vi "Slewing Test.vi"(8 "error in (no error)":errorcluster, 10 "Model in":refnum<class "Model.lvclass">, 11 "Test Actuator State in":refnum<class "Test Actuator State.lvclass">) -> (0 "error out":errorcluster, 2 "Model out":refnum<class "Model.lvclass">, 3 "Test Actuator State out":refnum<class "Test Actuator State.lvclass">)   [LabVIEW 2016, in "Test Actuator State.lvclass"]
uses:
  Test Actuator State.lvclass
  Model/Model/Model.lvclass
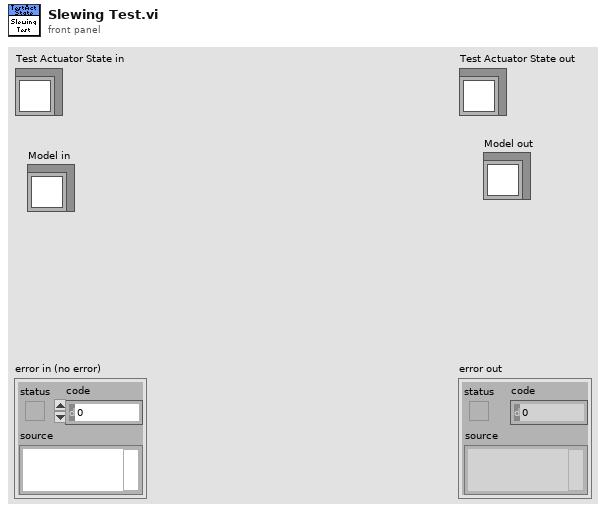
[diagram p1: front panel]
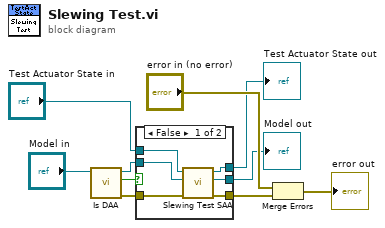
[diagram p0: block diagram]
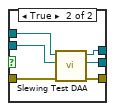
[diagram p2: hidden frame]
diagram:
  n1 = call "Is DAA.vi"("Model in"="Model in") -> ("error out"=w2:errorcluster, "IsDAA"=w7:bool, "Model out"=w6:refnum<class "Model.lvclass">)  [unwired: 8 in]
  n2 = case shown="False" w7 {
    tunnel: w6 -> [w14 w22]
    tunnel: "Test Actuator State in" -> [w16 w21]
    tunnel: [w15 w20] -> w4
    tunnel: [w13 w19] -> w3
    tunnel: w2 -> [w12 w18]
    tunnel: [w11 w17] -> w1
    frame False {
      n3 = call "Slewing Test SAA.vi"("error in (no error)"=w12, "Model in"=w14, "Test Actuator State in"=w16) -> ("error out"=w11:errorcluster, "Model out"=w13:refnum<class "Model.lvclass">, "Test Actuator State out"=w15:refnum<class "Test Actuator State.lvclass">)  [unwired: 6 in]
    }
    frame True {
      n4 = call "Slewing Test DAA.vi"("error in (no error)"=w18, "Model in"=w22, "Test Actuator State in"=w21) -> ("error out"=w17:errorcluster, "Model out"=w19:refnum<class "Model.lvclass">, "Test Actuator State out"=w20:refnum<class "Test Actuator State.lvclass">)  [unwired: 6 in]
    }
  }
  "Test Actuator State out" <- w4
  "Model out" <- w3
  n5 = Merge Errors("error in (no error)", w1) -> (→"error out":errorcluster)
